vi "CAN_Send Diag Message.vi"(0 "Write Session in":refnum<k21>, 1 "Read Session in":refnum<k21>, 2 "Parttype ref":refnum<vi>, 3 "ODX File Path":path=path "C:/LegacyApp/DB_0CA_7100_4M0_0004_73710BVW3710/DB_0CA_7100_4M0_0004_73710BVW3710/DB_0CA_7100_4M0_0004_73710BVW3710.odx", 4 "Tx Msg":u8[](array[numeric])=[2, 26, 156, 255, 255, 255, 255, 255] format="%02x", 5 "error in (no error)":errorcluster, 6 "Enum":T2=enum."Get Calibration Status", 7 "Download CAL Progress":refnum<vi>, 10 "Postion":u16=3, 11 "Download CAL Time":refnum<vi>, 12 "Autotest":bool, 14 "ECU Info in":T1, 17 "Tester":refnum<k21>) -> (13 "Response Good?":bool, 15 "ECU Info":T1, 16 "pass?":bool, 18 "TxRx Data":string[][](array[string]), 19 "error out":errorcluster)   [LabVIEW 2014]
uses:
  Diagnostic Message.ctl
  typedefs/parttype.ctl
  <vilib>/xnet/xnet.llb/XNET Frame CAN.ctl
  <vilib>/xnet/xnet.llb/XNET Frame Type CAN.ctl
  CAN Communication VI's/Typedefs/Select Session.ctl
  typedefs/All Motions.ctl
  <vilib>/xnet/xnet.llb/XNET Write (Frame CAN).vi
  <vilib>/xnet/xnet.llb/XNET Read (Frame CAN).vi
panel:
  out "Rx Message":u8[](array[numeric]) format="%02x"
  out "Error String Out":string
  in  "Tx Arbitration Id":u32=402391172 format="%.0x"
  out "Part Number":string
  out "Vehicle Type":string
  out "SW level":string
  out "Calibrated":bool
  out "HW level":string
  out "CAL level":string
  out "Boot level":string
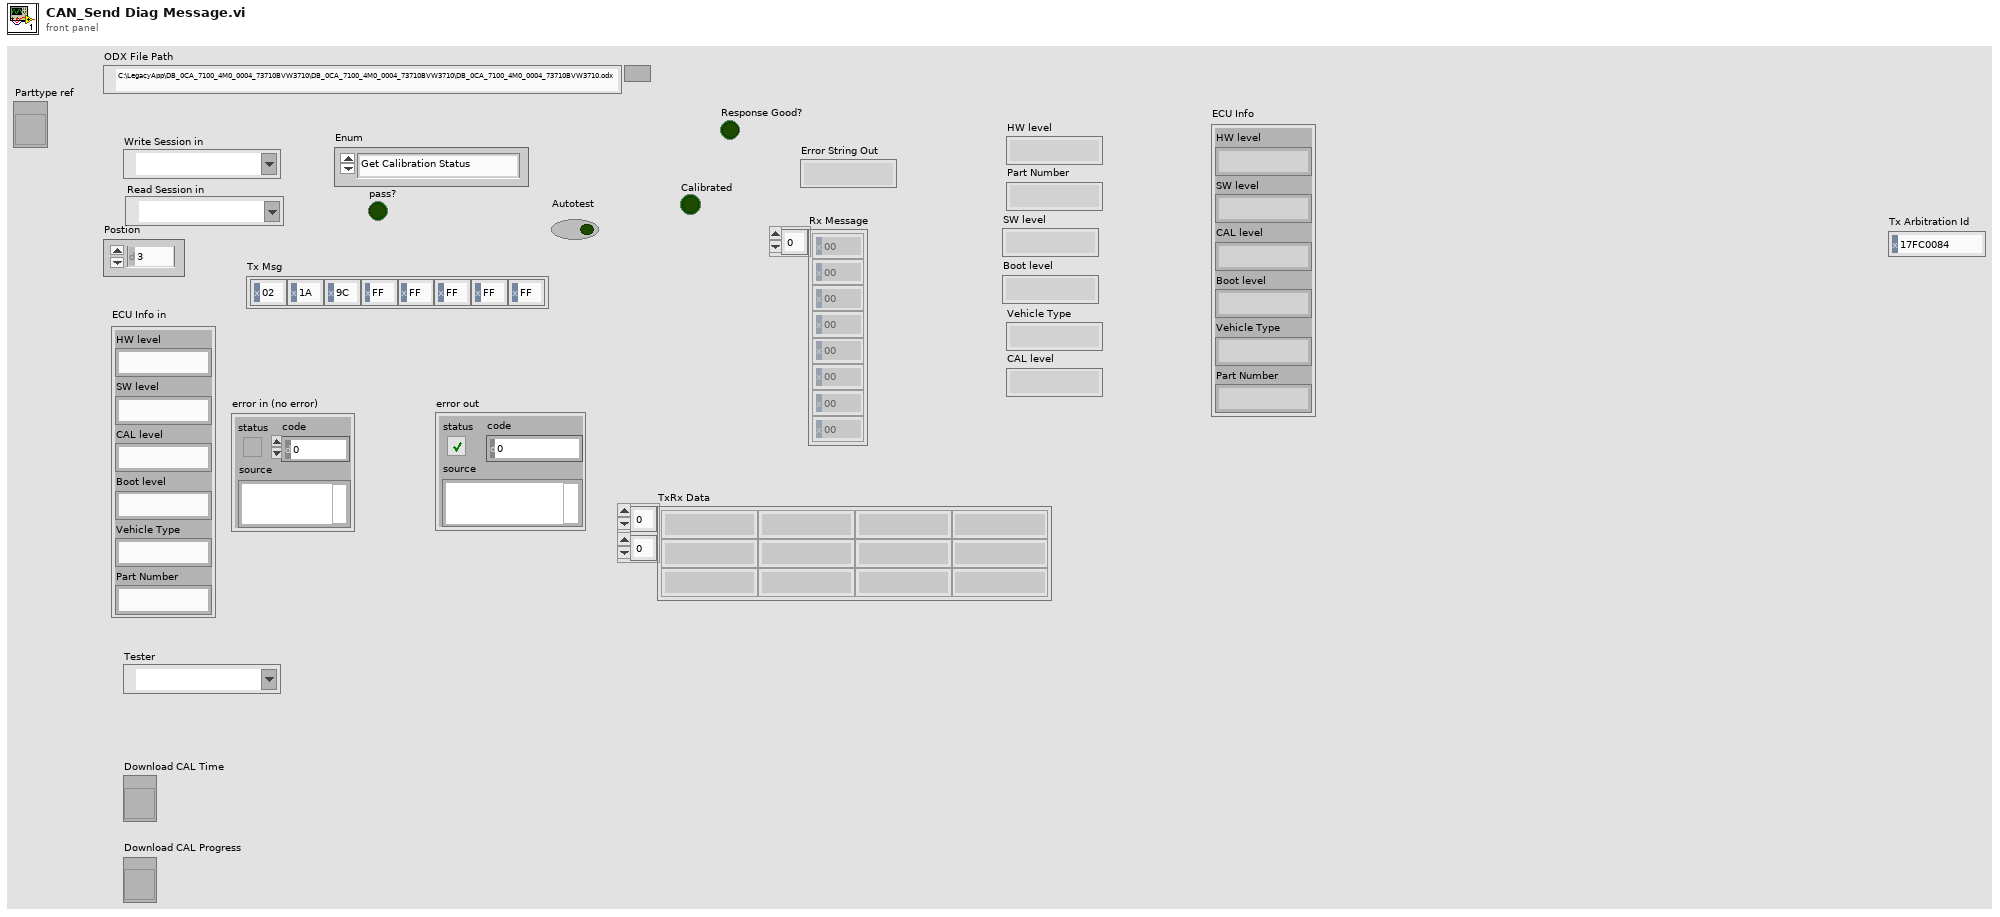
[diagram p1: front panel]
types:
  T1 = cluster{"HW level":string, "SW level":string, "CAL level":string, "Boot level":string, "Vehicle Type":string, "Part Number":string}
  T2 = typedef "Diagnostic Message.ctl" = enum16{"User Select", "Get User Multi-Frame", "Diag Session Prog", "Diag Session Ext", "Diag Session EOL", "Diag Session Default", "Diag Session Dev", "Read Active Session", "Read HW", "Read SW", "Read Part Number", "Learn Start Glass", "Learn Start Rollo", "Get Calibration Status", "Read SW CAL Boot", "Go to Position", "Get Parametric Mode Status", "Enable Parametric Mode", "Disable Parametric Mode", "Enable Production Mode", "Disable Production Mode", "Reset ECU", "Go to Slide Close", "Go to Slide Open", "Go to Vent Open", "Rollo Open", "Rollo Close", "Write Vehicle Type", "Read Vehicle Type", "Clear DTC", "Check Teach DTC", "Write Shop Code", "Download CAL", "Finish Flash", "Delete RP RF"}
  T3 = typedef "XNET Frame CAN.ctl" = cluster{"timestamp":timestamp, "payload":u8[], "identifier":u32, "type":T4, "extended?":bool, "echo?":bool}
  T4 = typedef "XNET Frame Type CAN.ctl" = u8
  T5 = typedef "Select Session.ctl" = enum16{"DefaultSession", "Development", "Extended", "EOL", "Programming"}
  T6 = typedef "All Motions.ctl" = enum16{"Idle", "Glass Teach", "Glass Slide Open", "Glass Slide Open 2", "Glass Slide Close", "Glass Slide Close 2", "Glass Vent Open", "Glass Vent Close", "Sunshade Teach", "Sunshade Teach 2", "Sunshade Open", "Sunshade Open 2", "Sunshade Close", "Sunshade Close 2", "Glass Slide Open Sunshade Open", "Glass Slide Open 2 Sunshade Open", "Glass Slide Open Sunshade Close", "Glass Slide Open 2 Sunshade Close", "Glass Slide Close Sunshade Open", "Glass Slide Close 2 Sunshade Open", "Glass Slide Close Sunshade Close", "Glass Slide Close 2 Sunshade Close", "Glass Vent Open Sunshade Open", "Glass Vent Open Sunshade Close", "Glass Vent Close Sunshade Open", "Glass Vent Close Sunshade Close", "Express Glass Slide Open", "Express Glass Slide Open 2", "Express Glass Slide Close", "Express Glass Slide Close 2", "Express Glass Vent Open", "Express Glass Vent Close", "Express Sunshade Open", "Express Sunshade Close", "Express Sunshade Open 2", "Express Sunshade Close 2", "Express Glass Slide Open Sunshade Open", "Express Glass Slide Open 2 Sunshade Open", "Express Glass Slide Open Sunshade Close", "Express Glass Slide Open 2 Sunshade Close", "Express Glass Slide Close Sunshade Open", "Express Glass Slide Close 2 Sunshade Open", "Express Glass Slide Close Sunshade Close", "Express Glass Slide Close 2 Sunshade Close", "Express Glass Vent Open Sunshade Open", "Express Glass Vent Open Sunshade Close", "Express Glass Vent Close Sunshade Open", "Express Glass Vent Close Sunshade Close", "Goto Position Glass", "Goto Position Sunshade"}
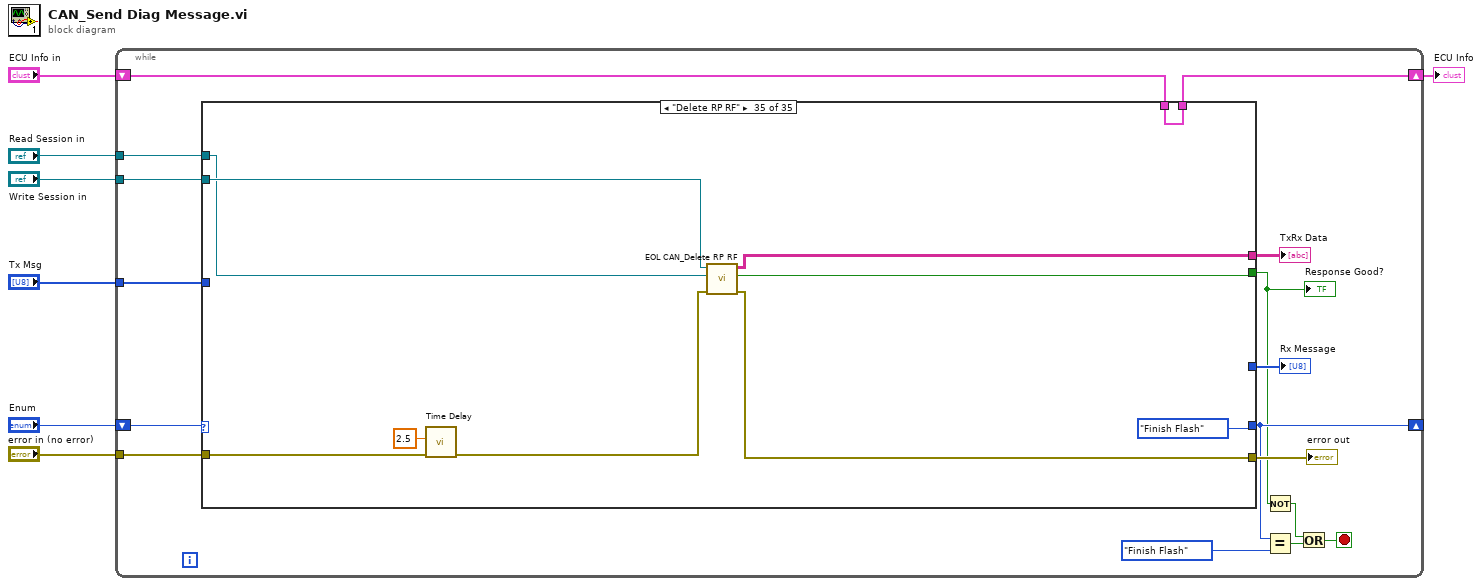
[diagram p0: block diagram]
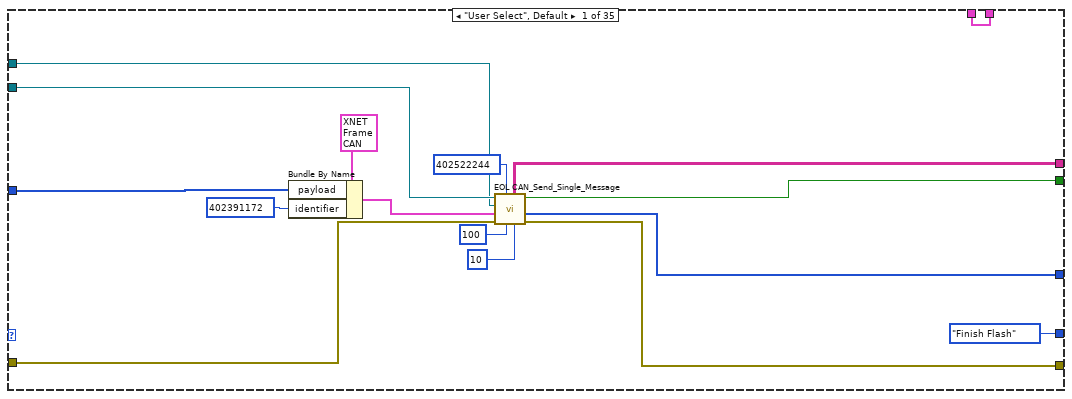
[diagram p2: hidden frame]
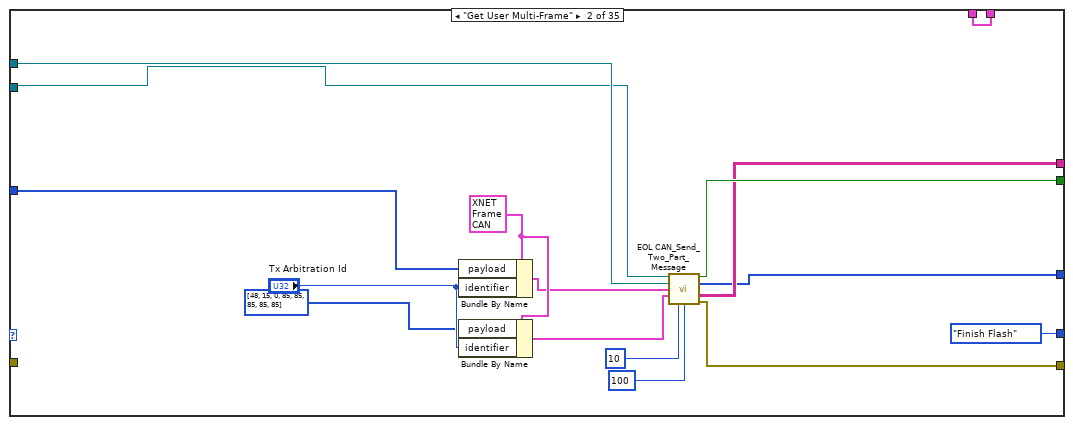
[diagram p3: hidden frame]
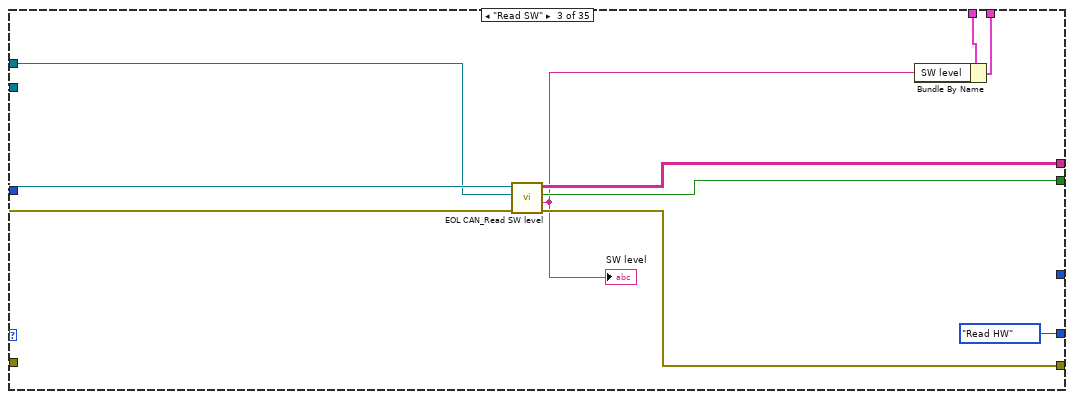
[diagram p4: hidden frame]
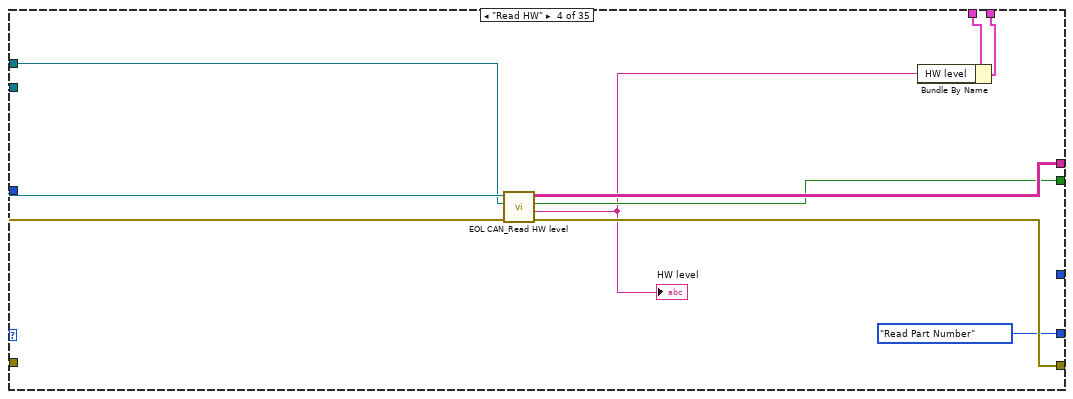
[diagram p5: hidden frame]
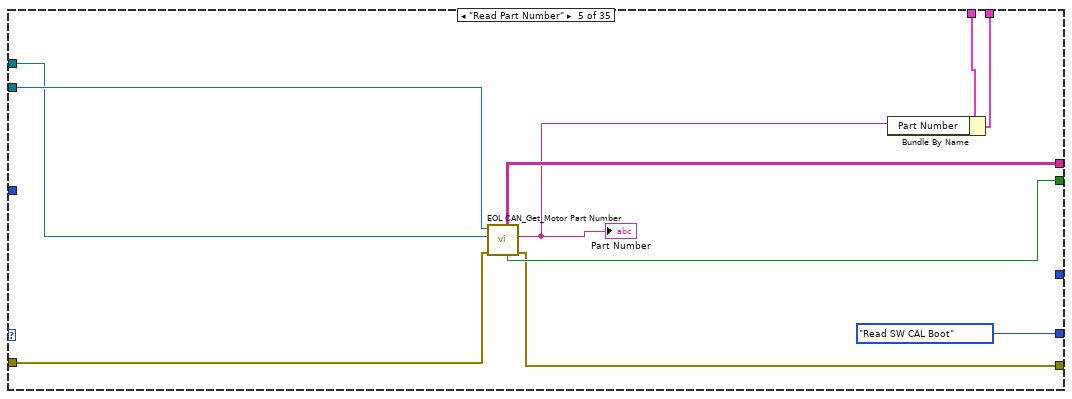
[diagram p6: hidden frame]
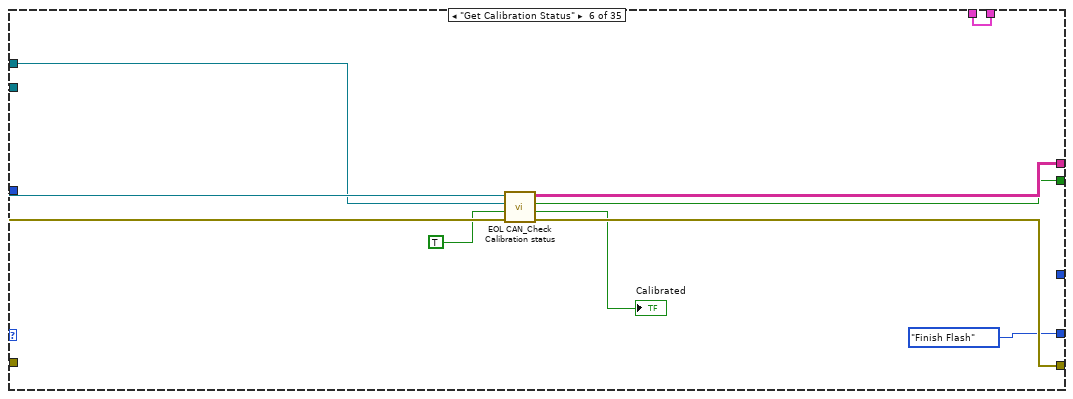
[diagram p7: hidden frame]
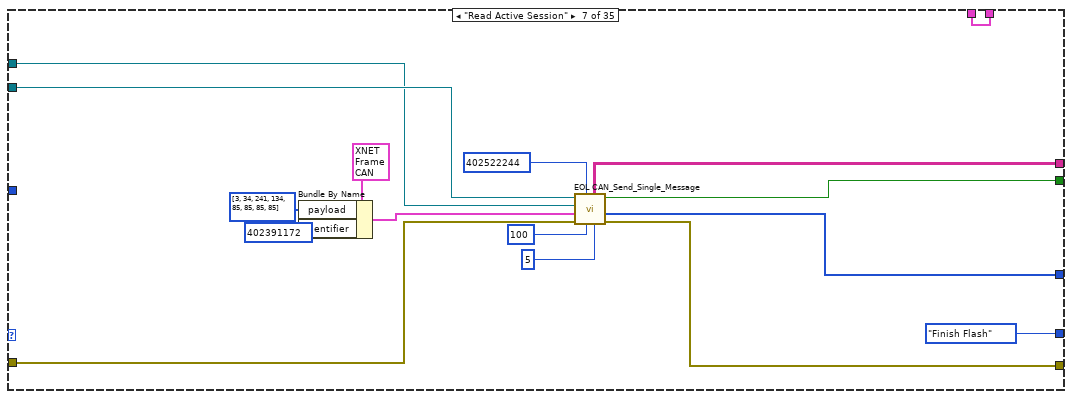
[diagram p8: hidden frame]
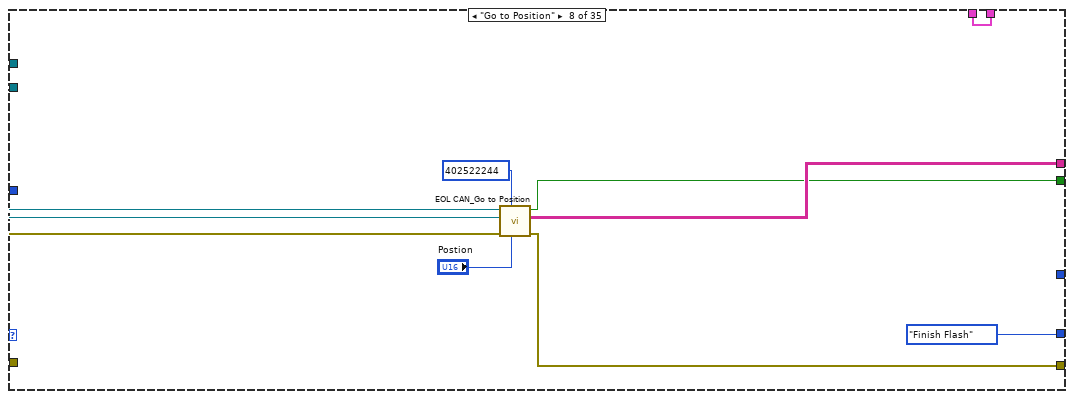
[diagram p9: hidden frame]
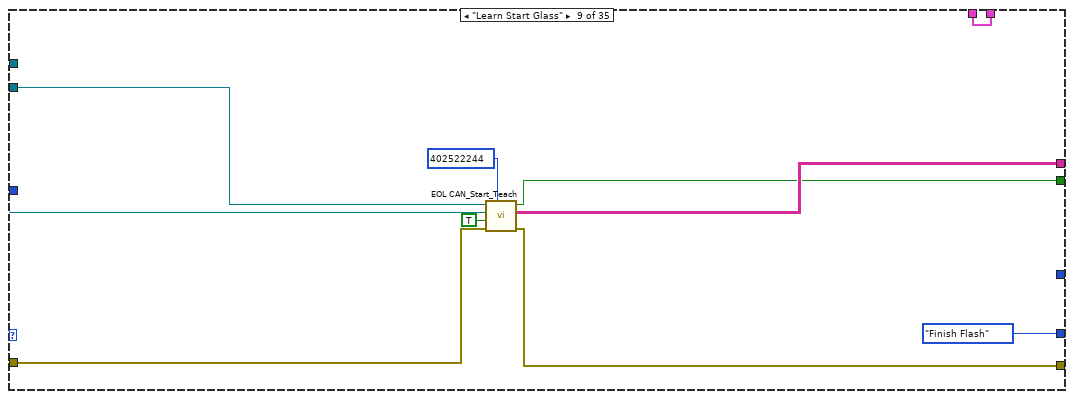
[diagram p10: hidden frame]
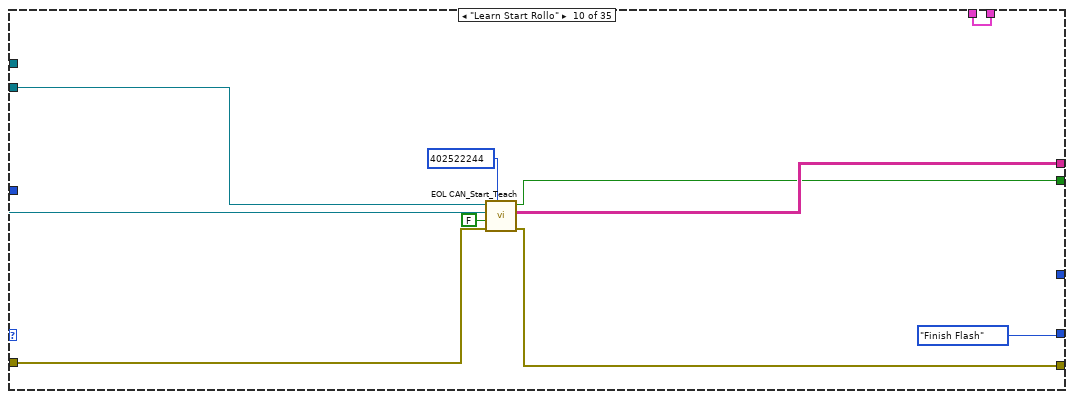
[diagram p11: hidden frame]
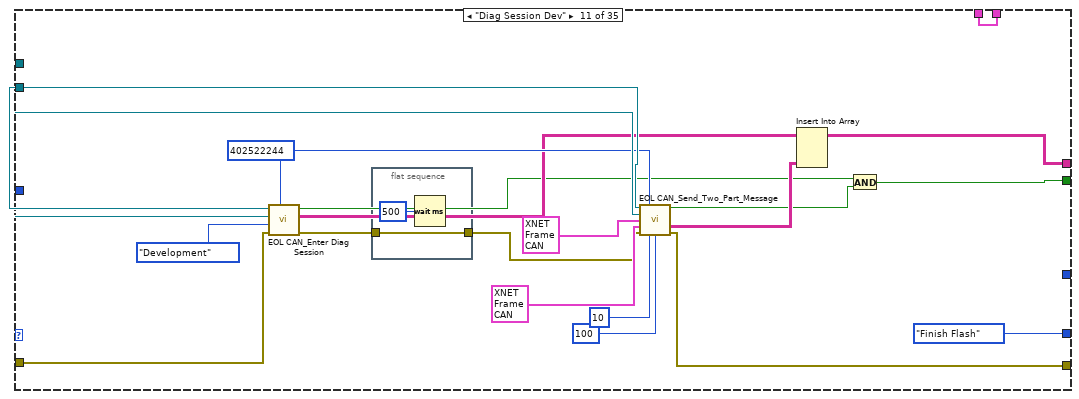
[diagram p12: hidden frame]
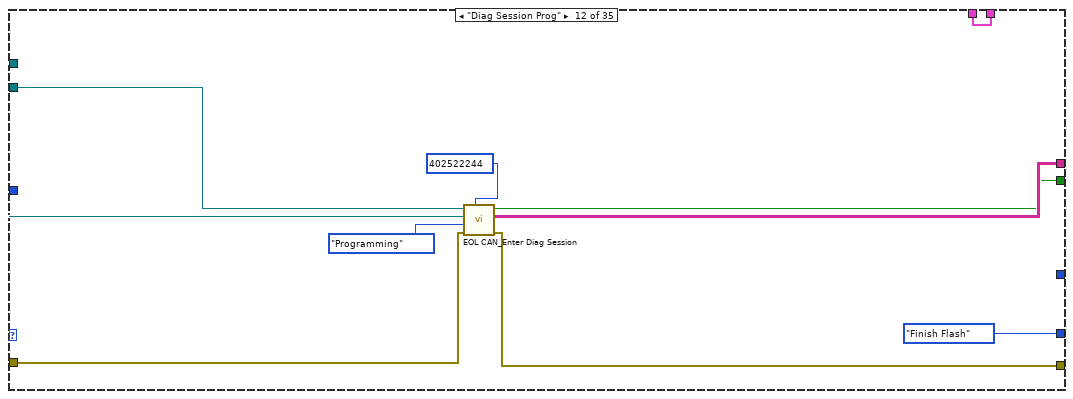
[diagram p13: hidden frame]
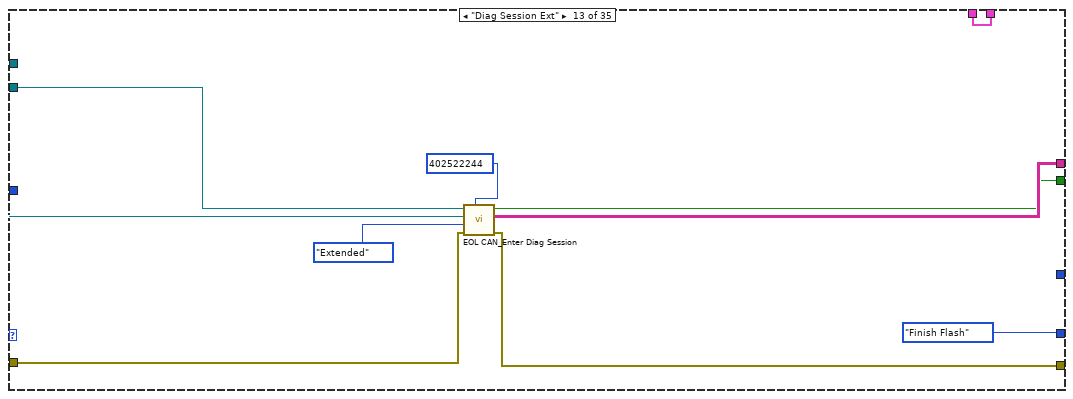
[diagram p14: hidden frame]
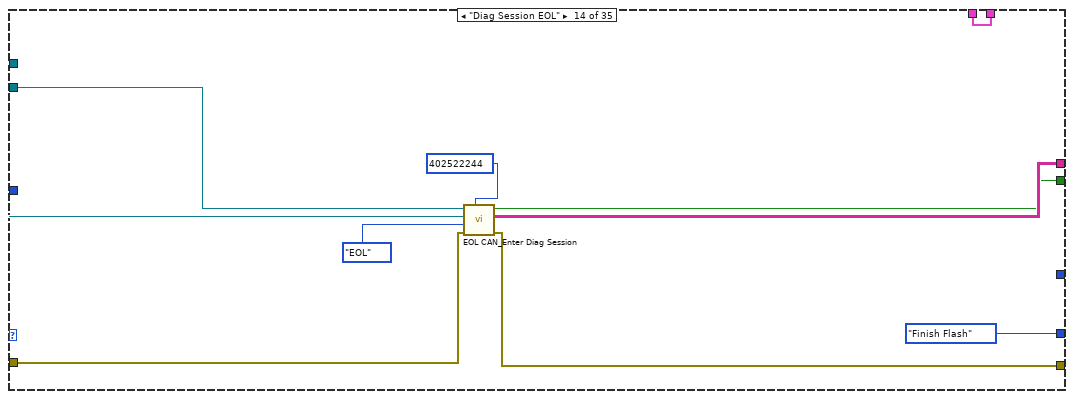
[diagram p15: hidden frame]
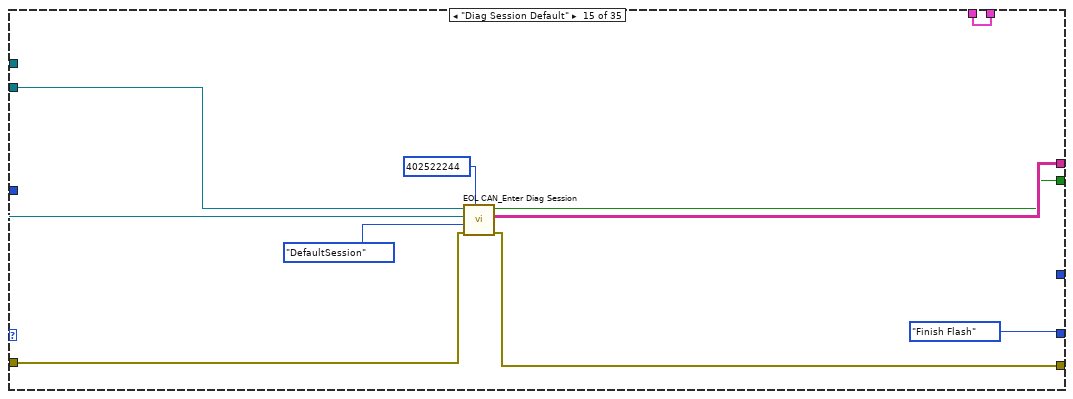
[diagram p16: hidden frame]
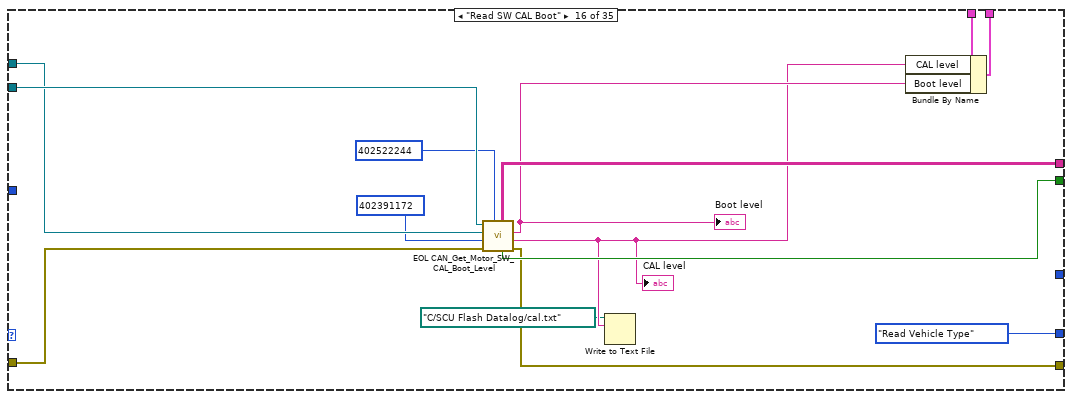
[diagram p17: hidden frame]
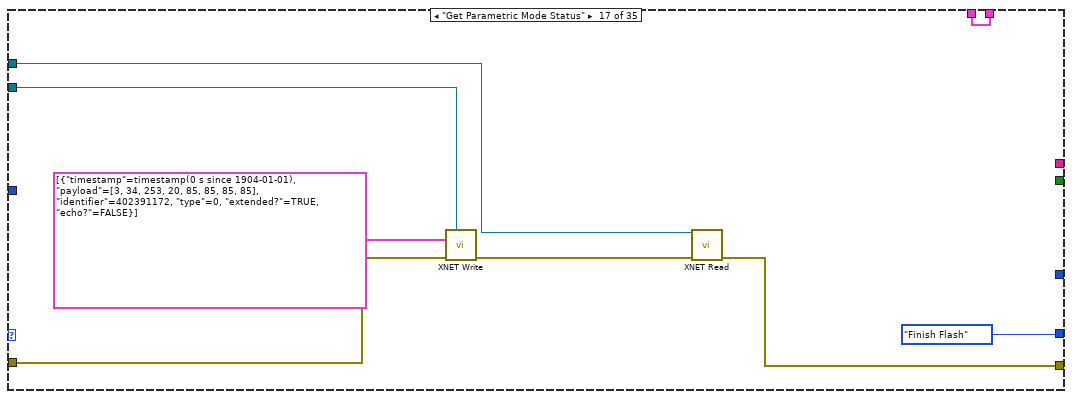
[diagram p18: hidden frame]
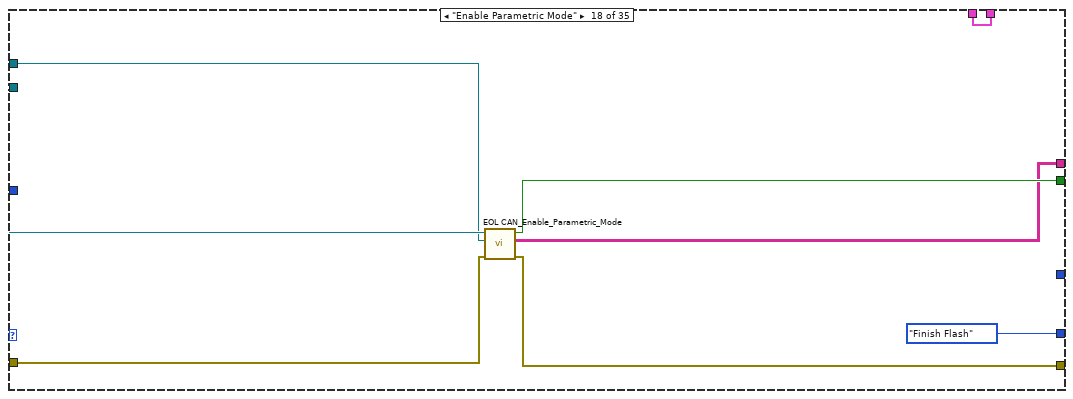
[diagram p19: hidden frame]
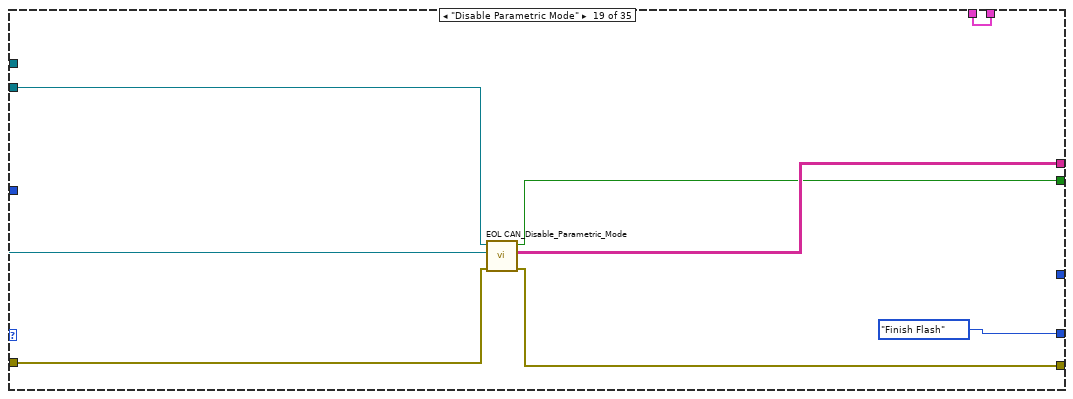
[diagram p20: hidden frame]
diagram:
  n1 = while {
    tunnel: "error in (no error)" -> [w23]
    tunnel: "Read Session in" -> [w21]
    tunnel: "Write Session in" -> [w20]
    shift-right: [w17] -> w3
    shift-left: "ECU Info in" -> [w16]
    tunnel: "Tx Msg" -> [w15]
    shift-right: [w10] -> _
    shift-left: "Enum" -> [w19]
    stop <- w13 stop-if-true
    n2 = case shown="\"Delete RP RF\"" w19 {
      tunnel: w21 -> [w38 w47 w60 w70 w83 w94 w110 w118 w129 w139 w157 w167 w177 w187 w197 w215 w223 w231 w236 w247 w255 w264 w274 w284 w294 w304 w314 w318 w326 w350 w365 w372 w382 _ w411]
      tunnel: w20 -> [w39 w46 w61 w71 w84 w95 w111 w119 w130 w140 w159 w168 w178 w188 w198 w216 w225 w232 w237 w248 w256 w265 w275 w285 w295 w305 w315 w319 w327 w351 w364 w373 w384 _ w412]
      tunnel: w23 -> [w37 _ w65 w75 w85 w93 w109 w121 w131 w141 w161 w173 w183 w193 w203 w217 w224 w233 w241 w249 w257 w266 w276 w286 w296 w306 w316 _ _ _ w366 w374 w383 w402 w406]
      tunnel: [w36 w42 w64 w74 w80 w92 w108 w120 w127 w137 w158 w172 w182 w192 w202 w210 w220 w228 w240 w244 w252 w260 w270 w280 w290 w300 w310 w322 w330 errorcluster {"status"=FALSE, "code"=0, "source"=""} ("error IO") w359 w371 w381 w402 w408] -> w22
      tunnel: [w35 w43 w63 w73 w82 w91 w107 w116 w126 w136 w151 w171 w181 w191 w201 w212 _ w229 w239 w245 w253 w262 w271 w281 w291 w301 w311 w323 w331 w346 w361 w369 _ _ w410] -> w18
      tunnel: [w34 w44 w62 w72 w81 w88 w106 w115 w125 w135 w148 w170 w180 w190 w200 w211 _ w230 w238 w246 w254 w261 w272 w282 w292 w302 w312 w321 w329 w336 w360 w370 _ _ w409] -> w9
      tunnel: [w33 w41 _ _ _ _ w103 _ _ _ _ _ _ _ _ _ _ _ _ _ _ _ _ _ _ _ _ w320 w328 _ _ _ _ _ _] -> w14
      tunnel: [w26 w55 w58 w67 w78 w87 w97 w113 w124 w134 w143 w165 w175 w185 w195 w208 w219 w227 w235 w243 w251 w259 w268 w278 w288 w298 w308 w324 w332 w354 w357 w368 w376 w403 w413] -> w17
      tunnel: w16 -> [w26 w55 w59 w68 w77 w87 w97 w113 w124 w134 w143 w165 w175 w185 w195 w209 w219 w227 w235 w243 w251 w259 w268 w278 w288 w298 w308 w324 w332 w354 w358 w368 w376 w403 w413]
      tunnel: w15 -> [w25 w45 _ _ _ _ _ _ _ _ _ _ _ _ _ _ _ _ _ _ _ _ _ _ _ _ _ _ _ _ _ _ _ _ _]
      tunnel: [Diagnostic_Message."Finish Flash" ("Enum") Diagnostic_Message."Finish Flash" ("Enum") Diagnostic_Message."Read HW" ("Enum") Diagnostic_Message."Read Part Number" ("Enum") Diagnostic_Message."Read SW CAL Boot" ("Enum") Diagnostic_Message."Finish Flash" ("Enum") Diagnostic_Message."Finish Flash" ("Enum") Diagnostic_Message."Finish Flash" ("Enum") Diagnostic_Message."Finish Flash" ("Enum") Diagnostic_Message."Finish Flash" ("Enum") Diagnostic_Message."Finish Flash" ("Enum") Diagnostic_Message."Finish Flash" ("Enum") Diagnostic_Message."Finish Flash" ("Enum") Diagnostic_Message."Finish Flash" ("Enum") Diagnostic_Message."Finish Flash" ("Enum") Diagnostic_Message."Read Vehicle Type" ("Enum") Diagnostic_Message."Finish Flash" ("Enum") Diagnostic_Message."Finish Flash" ("Enum") Diagnostic_Message."Finish Flash" ("Enum") Diagnostic_Message."Delete RP RF" ("Enum") Diagnostic_Message."Finish Flash" ("Enum") Diagnostic_Message."Finish Flash" ("Enum") Diagnostic_Message."Finish Flash" ("Enum") Diagnostic_Message."Finish Flash" ("Enum") Diagnostic_Message."Finish Flash" ("Enum") Diagnostic_Message."Finish Flash" ("Enum") Diagnostic_Message."Finish Flash" ("Enum") Diagnostic_Message."Finish Flash" ("Enum") Diagnostic_Message."Finish Flash" ("Enum") w339 Diagnostic_Message."Enable Production Mode" ("Enum") Diagnostic_Message."Finish Flash" ("Enum") Diagnostic_Message."Finish Flash" ("Enum") Diagnostic_Message."Finish Flash" ("Enum") Diagnostic_Message."Finish Flash" ("Enum")] -> w10
      frame "User Select", Default {
        n3 = Bundle By Name(cluster=T3 {"timestamp"=timestamp(0 s since 1904-01-01), "payload"=[2, 39, 3, 85, 85, 85, 85, 85], "identifier"=402391172, "type"=0, "extended?"=TRUE, "echo?"=FALSE} ("Tx CAN frame"), "payload"=w25, "identifier"=u32 402391172) -> (w31:T3)
        n4 = call "EOL CAN_Send_Single_Message.vi"("Retries"=10, "Msg Wait Time"=u32 100, "Rx Arbitration Id"=u32 402522244, "Error in"=w37, "Tx CAN frame"=w31, "Read Session in"=w38, "Write Session in"=w39) -> ("Error out"=w36:errorcluster, "Rx Message"=w33:u8[], "Response Good?"=w34:bool, "TxRx Data"=w35:string[][])  [unwired: 1 out]
      }
      frame "Get User Multi-Frame" {
        w49 = T3 {"timestamp"=timestamp(0 s since 1904-01-01), "payload"=[2, 39, 3, 85, 85, 85, 85, 85], "identifier"=402391172, "type"=0, "extended?"=TRUE, "echo?"=FALSE} ("Tx CAN frame 1")
        n5 = Bundle By Name(cluster=w49, "payload"=w45, "identifier"="Tx Arbitration Id") -> (w48:T3)
        n6 = Bundle By Name(cluster=w49, "payload"=u8[] [48, 15, 0, 85, 85, 85, 85, 85] ("Transmit Data"), "identifier"="Tx Arbitration Id") -> (w50:T3)
        n7 = call "EOL CAN_Send_Two_Part_Message.vi"("Write Session in"=w46, "Read Session in"=w47, "Tx CAN frame 1"=w48, "Tx CAN frame 2"=w50, "Retries"=10, "Msg Wait Time"=u32 100) -> ("Response Good?"=w44:bool, "Rx Data"=w41:u8[], "TxRx Data"=w43:string[][], "error out"=w42:errorcluster)  [unwired: 6 in]
      }
      frame "Read SW" {
        n8 = call "EOL CAN_Read SW level.vi"("error in (no error)"=w65, "Read Session in"=w60, "Write Session in"=w61) -> ("error out"=w64:errorcluster, "SW level"=w57:string, "Response Good?"=w62:bool, "TxRx Data"=w63:string[][])  [unwired: 5 in]
        "SW level" <- w57
        n9 = Bundle By Name(cluster=w59, "SW level"=w57) -> (w58:T1)
      }
      frame "Read HW" {
        n10 = call "EOL CAN_Read HW level.vi"("error in (no error)"=w75, "Read Session in"=w70, "Write Session in"=w71) -> ("error out"=w74:errorcluster, "HW level"=w69:string, "Response Good?"=w72:bool, "TxRx Data"=w73:string[][])  [unwired: 5 in]
        "HW level" <- w69
        n11 = Bundle By Name(cluster=w68, "HW level"=w69) -> (w67:T1)
      }
      frame "Read Part Number" {
        n12 = call "EOL CAN_Get_Motor Part Number.vi"("error in (no error)"=w85, "Read Session in"=w83, "Write Session in"=w84) -> ("error out"=w80:errorcluster, "Part Number"=w79:string, "Response Good?"=w81:bool, "TxRx Data"=w82:string[][])  [unwired: 5 in]
        "Part Number" <- w79
        n13 = Bundle By Name(cluster=w77, "Part Number"=w79) -> (w78:T1)
      }
      frame "Get Calibration Status" {
        n14 = call "EOL CAN_Check Calibration status.vi"("error in (no error)"=w93, "Glass?"=TRUE, "Read Session in"=w94, "Write Session in"=w95) -> ("error out"=w92:errorcluster, "Calibrated"=→"Calibrated":bool, "Response Good?"=w88:bool, "TxRx Data"=w91:string[][])  [unwired: 4 in]
      }
      frame "Read Active Session" {
        n15 = Bundle By Name(cluster=T3 {"timestamp"=timestamp(0 s since 1904-01-01), "payload"=[2, 39, 3, 85, 85, 85, 85, 85], "identifier"=402391172, "type"=0, "extended?"=TRUE, "echo?"=FALSE} ("Tx CAN frame"), "payload"=u8[] [3, 34, 241, 134, 85, 85, 85, 85], "identifier"=u32 402391172) -> (w100:T3)
        n16 = call "EOL CAN_Send_Single_Message.vi"("Retries"=5, "Msg Wait Time"=u32 100, "Rx Arbitration Id"=u32 402522244, "Error in"=w109, "Tx CAN frame"=w100, "Read Session in"=w110, "Write Session in"=w111) -> ("Error out"=w108:errorcluster, "Rx Message"=w103:u8[], "Response Good?"=w106:bool, "TxRx Data"=w107:string[][])  [unwired: 1 out]
      }
      frame "Go to Position" {
        n17 = call "EOL CAN_Go to Position.vi"("Postion"="Postion", "Rx Arbitration Id"=u32 402522244, "Error in"=w121, "Read Session in"=w118, "Write Session in"=w119) -> ("Error out"=w120:errorcluster, "TxRx Data"=w116:string[][], "Response Good?"=w115:bool)  [unwired: 4 in]
      }
      frame "Learn Start Glass" {
        n18 = call "EOL CAN_Start_Teach.vi"("Rx Arbitration Id"=u32 402522244, "Error in"=w131, "Glass?"=TRUE, "Read Session in"=w129, "Write Session in"=w130) -> ("Error out"=w127:errorcluster, "TxRx Data"=w126:string[][], "Response Good?"=w125:bool)  [unwired: 4 in]
      }
      frame "Learn Start Rollo" {
        n19 = call "EOL CAN_Start_Teach.vi"("Rx Arbitration Id"=u32 402522244, "Error in"=w141, "Glass?"=FALSE, "Read Session in"=w139, "Write Session in"=w140) -> ("Error out"=w137:errorcluster, "TxRx Data"=w136:string[][], "Response Good?"=w135:bool)  [unwired: 4 in]
      }
      frame "Diag Session Dev" {
        w156 = u32 402522244 ("Rx Arbitration Id")
        n20 = call "EOL CAN_Enter Diag Session.vi"("Rx Arbitration Id"=w156, "Error in"=w161, "Session"=Select_Session."Development", "Read Session in"=w157, "Write Session in"=w159) -> ("Error out"=w147:errorcluster, "TxRx Data"=w153:string[][], "Response Good?"=w149:bool)  [unwired: 4 in]
        n21 = flat-sequence {
          tunnel: w147 -> [w162]
          tunnel: [w162] -> w146
          frame #0 {
            n22 = Wait (ms)(milliseconds to wait=u32 500) -> ()  [unwired: 1 out]
          }
        }
        n23 = call "EOL CAN_Send_Two_Part_Message.vi"("Write Session in"=w159, "Rx Arbitration Id"=w156, "Read Session in"=w157, "Tx CAN frame 1"=T3 {"timestamp"=timestamp(0 s since 1904-01-01), "payload"=[3, 34, 254, 253, 85, 85, 85, 85], "identifier"=402391172, "type"=8, "extended?"=TRUE, "echo?"=FALSE}, "Tx CAN frame 2"=T3 {"timestamp"=timestamp(0 s since 1904-01-01), "payload"=[48, 15, 0, 85, 85, 85, 85, 85], "identifier"=402391172, "type"=8, "extended?"=TRUE, "echo?"=FALSE}, "error in (no error)"=w146, "Retries"=10, "Msg Wait Time"=u32 100) -> ("Response Good?"=w150:bool, "TxRx Data"=w152:string[][], "error out"=w158:errorcluster)  [unwired: 4 in, 1 out]
        n24 = Insert Into Array(array=w153, new element=w152) -> (w151:string[][])  [unwired: 2 in]
        n25 = And(x=w149, y=w150) -> (x .and. y?=w148:bool)
      }
      frame "Diag Session Prog" {
        n26 = call "EOL CAN_Enter Diag Session.vi"("Rx Arbitration Id"=u32 402522244, "Error in"=w173, "Session"=Select_Session."Programming", "Read Session in"=w167, "Write Session in"=w168) -> ("Error out"=w172:errorcluster, "TxRx Data"=w171:string[][], "Response Good?"=w170:bool)  [unwired: 4 in]
      }
      frame "Diag Session Ext" {
        n27 = call "EOL CAN_Enter Diag Session.vi"("Rx Arbitration Id"=u32 402522244, "Error in"=w183, "Session"=Select_Session."Extended", "Read Session in"=w177, "Write Session in"=w178) -> ("Error out"=w182:errorcluster, "TxRx Data"=w181:string[][], "Response Good?"=w180:bool)  [unwired: 4 in]
      }
      frame "Diag Session EOL" {
        n28 = call "EOL CAN_Enter Diag Session.vi"("Rx Arbitration Id"=u32 402522244, "Error in"=w193, "Session"=Select_Session."EOL", "Read Session in"=w187, "Write Session in"=w188) -> ("Error out"=w192:errorcluster, "TxRx Data"=w191:string[][], "Response Good?"=w190:bool)  [unwired: 4 in]
      }
      frame "Diag Session Default" {
        n29 = call "EOL CAN_Enter Diag Session.vi"("Rx Arbitration Id"=u32 402522244, "Error in"=w203, "Session"=Select_Session."DefaultSession", "Read Session in"=w197, "Write Session in"=w198) -> ("Error out"=w202:errorcluster, "TxRx Data"=w201:string[][], "Response Good?"=w200:bool)  [unwired: 4 in]
      }
      frame "Read SW CAL Boot" {
        n30 = call "EOL CAN_Get_Motor_SW_CAL_Boot_Level.vi"("Rx Arbitration Id"=u32 402522244, "error in (no error)"=w217, "Tx Arbitration Id"=u32 402391172 ("identifier"), "Read Session in"=w215, "Write Session in"=w216) -> ("error out"=w210:errorcluster, "CAL level"=w205:string, "Boot level"=w207:string, "Response Good?"=w211:bool, "TxRx Data"=w212:string[][])  [unwired: 1 in, 1 out]
        "Boot level" <- w207
        "CAL level" <- w205
        n31 = Write to Text File(file (use dialog)=path "C:/SCU Flash Datalog/cal.txt", text=w205) -> ()  [unwired: 2 in, 3 out]
        n32 = Bundle By Name(cluster=w209, "CAL level"=w205, "Boot level"=w207) -> (w208:T1)
      }
      frame "Get Parametric Mode Status" {
        n33 = call-poly <vilib>:"XNET Write.vi"("session in"=w225, "data"=T3[] [{"timestamp"=timestamp(0 s since 1904-01-01), "payload"=[3, 34, 253, 20, 85, 85, 85, 85], "identifier"=402391172, "type"=0, "extended?"=TRUE, "echo?"=FALSE}] ("Frame to Send 2"), "error in (no error)"=w224) -> ("error out"=w221:errorcluster)  [unwired: 11 in, 1 out]
        n34 = call-poly <vilib>:"XNET Read.vi"("session in"=w223, "error in (no error)"=w221) -> ("error out"=w220:errorcluster)  [unwired: 10 in, 3 out]
      }
      frame "Enable Parametric Mode" {
        n35 = call "EOL CAN_Enable_Parametric_Mode.vi"("Error in"=w233, "Read Session in"=w231, "Write Session in"=w232) -> ("Error out"=w228:errorcluster, "debug log"=w229:string[][], "Response Good?"=w230:bool)  [unwired: 6 in]
      }
      frame "Disable Parametric Mode" {
        n36 = call "EOL CAN_Disable_Parametric_Mode.vi"("Error in"=w241, "Read Session in"=w236, "Write Session in"=w237) -> ("Error out"=w240:errorcluster, "debug log"=w239:string[][], "Response Good?"=w238:bool)  [unwired: 6 in]
      }
      frame "Enable Production Mode" {
        n37 = call "EOL CAN_Enable_Production_Mode.vi"("Error in"=w249, "Read Session in"=w247, "Write Session in"=w248) -> ("Error out"=w244:errorcluster, "debug log"=w245:string[][], "Response Good?"=w246:bool)  [unwired: 6 in]
      }
      frame "Disable Production Mode" {
        n38 = call "EOL CAN_Disable_Production_Mode.vi"("Error in"=w257, "Read Session in"=w255, "Write Session in"=w256) -> ("Error out"=w252:errorcluster, "debug log"=w253:string[][], "Response Good?"=w254:bool)  [unwired: 6 in]
      }
      frame "Reset ECU" {
        n39 = call "EOL CAN_Reset ECU.vi"("Rx Arbitration Id"=u32 402522244, "Error in"=w266, "Read Session in"=w264, "Write Session in"=w265) -> ("Error out"=w260:errorcluster, "Response Good?"=w261:bool, "TxRx Data"=w262:string[][])  [unwired: 5 in]
      }
      frame "Go to Slide Close" {
        n40 = call "EOL CAN_Target Motion.vi"("Rx Arbitration Id"=u32 402522244, "Error in"=w276, "All Motions"=All_Motions."Glass Slide Close", "Read Session in"=w274, "Write Session in"=w275) -> ("Error out"=w270:errorcluster, "TxRx Data"=w271:string[][], "Response Good?"=w272:bool)  [unwired: 4 in]
      }
      frame "Go to Slide Open" {
        n41 = call "EOL CAN_Target Motion.vi"("Rx Arbitration Id"=u32 402522244, "Error in"=w286, "All Motions"=All_Motions."Glass Slide Open", "Read Session in"=w284, "Write Session in"=w285) -> ("Error out"=w280:errorcluster, "TxRx Data"=w281:string[][], "Response Good?"=w282:bool)  [unwired: 4 in]
      }
      frame "Go to Vent Open" {
        n42 = call "EOL CAN_Target Motion.vi"("Rx Arbitration Id"=u32 402522244, "Error in"=w296, "All Motions"=All_Motions."Glass Vent Open", "Read Session in"=w294, "Write Session in"=w295) -> ("Error out"=w290:errorcluster, "TxRx Data"=w291:string[][], "Response Good?"=w292:bool)  [unwired: 4 in]
      }
      frame "Rollo Open" {
        n43 = call "EOL CAN_Target Motion.vi"("Rx Arbitration Id"=u32 402522244, "Error in"=w306, "All Motions"=All_Motions."Sunshade Open", "Read Session in"=w304, "Write Session in"=w305) -> ("Error out"=w300:errorcluster, "TxRx Data"=w301:string[][], "Response Good?"=w302:bool)  [unwired: 4 in]
      }
      frame "Rollo Close" {
        n44 = call "EOL CAN_Target Motion.vi"("Rx Arbitration Id"=u32 402522244, "Error in"=w316, "All Motions"=All_Motions."Sunshade Close", "Read Session in"=w314, "Write Session in"=w315) -> ("Error out"=w310:errorcluster, "TxRx Data"=w311:string[][], "Response Good?"=w312:bool)  [unwired: 4 in]
      }
      frame "Write Vehicle Type" {
        n45 = call "EOL CAN_Write Vehicle Type.vi"("Read Session in"=w318, "Write Session in"=w319) -> ("error out"=w322:errorcluster, "Rx Message"=w320:u8[], "Response Good?"=w321:bool, "Array"=w323:string[][])  [unwired: 6 in]
      }
      frame "Write Shop Code" {
        n46 = call "EOL CAN_Write Repair Shop Code.vi"("Read Session in"=w326, "Write Session in"=w327) -> ("error out"=w330:errorcluster, "Rx Message"=w328:u8[], "Response Good?"=w329:bool, "TxRxData"=w331:string[][])  [unwired: 6 in]
      }
      frame "Download CAL" {
        n47 = call "EOL CAN_Download CAL.vi"("DSC Write Session in"=w351, "Tester"="Tester", "Download CAL Time"="Download CAL Time", "Read Session in"=w350, "Parttype ref"="Parttype ref", "Glass?"=TRUE, "ODX File Path"="ODX File Path", "Download CAL Progress"="Download CAL Progress") -> ("Response Good?"=w336:bool, "TxRx Data"=w346:string[][], "Error String Out"=→"Error String Out":string, "fail"=w337:bool)  [unwired: 4 in]
        n48 = Not(x=w337) -> (.not. x?=w335:bool)
        n49 = Select(t=Diagnostic_Message."Read SW" ("Enum"), s="Autotest", f=Diagnostic_Message."Finish Flash" ("Enum")) -> (s? t:f=w340:T2)
        n50 = And(x=w336, y=w335) -> (x .and. y?=→"pass?":bool)
        n51 = Select(t=w340, s=w336, f=Diagnostic_Message."Finish Flash") -> (s? t:f=w339:T2)
      }
      frame "Read Vehicle Type" {
        n52 = call "EOL CAN_Get Vehicle type.vi"("Rx Arbitration Id"=u32 402522244, "error in (no error)"=w366, "Tx Arbitration Id"=u32 402391172, "Read Session in"=w365, "Write Session in"=w364) -> ("error out"=w359:errorcluster, "Vehicle Type"=w356:string, "Response Good?"=w360:bool, "TxRx Data"=w361:string[][])  [unwired: 3 in]
        "Vehicle Type" <- w356
        n53 = Bundle By Name(cluster=w358, "Vehicle Type"=w356) -> (w357:T1)
      }
      frame "Clear DTC" {
        n54 = call "EOL CAN_Clear_DTC's.vi"("Error in"=w374, "Read Session in"=w372, "Write Session in"=w373) -> ("Error out"=w371:errorcluster, "TxRx Data"=w369:string[][], "Response Good?"=w370:bool)  [unwired: 6 in]
      }
      frame "Check Teach DTC" {
        n55 = stacked-sequence {
          tunnel: w384 -> [w392 w400]
          tunnel: w383 -> [w391 w399]
          tunnel: [w389 _] -> w380
          tunnel: w382 -> [w390 w398]
          tunnel: [w388 _] -> w378
          tunnel: [_ w397] -> w377
          tunnel: [_ w396] -> w379
          frame #0 {
            n56 = call-poly <vilib>:"XNET Write.vi"("session in"=w392, "data"=T3[] [{"timestamp"=timestamp(0 s since 1904-01-01), "payload"=[2, 16, 79, 85, 85, 85, 85, 85], "identifier"=402391172, "type"=0, "extended?"=TRUE, "echo?"=FALSE}] ("Frame to Send 2"), "error in (no error)"=w391) -> ("error out"=w386:errorcluster)  [unwired: 11 in, 1 out]
            n57 = call "Time Delay22"("error in (no error)"=w386, "Delay Time (s)"=0.05) -> ("error out"=w385:errorcluster)  [unwired: 9 in]
            n58 = call-poly <vilib>:"XNET Read.vi"("session in"=w390, "error in (no error)"=w385) -> ("data"=w388:T3[], "error out"=w389:errorcluster)  [unwired: 10 in, 2 out]
          }
          frame #1 {
            n59 = call-poly <vilib>:"XNET Write.vi"("session in"=w400, "data"=T3[] [{"timestamp"=timestamp(0 s since 1904-01-01), "payload"=[3, 34, 241, 134, 85, 85, 85, 85], "identifier"=402391172, "type"=0, "extended?"=TRUE, "echo?"=FALSE}] ("Frame to Send 2"), "error in (no error)"=w399) -> ("error out"=w395:errorcluster)  [unwired: 11 in, 1 out]
            n60 = call-poly <vilib>:"XNET Read.vi"("session in"=w398, "error in (no error)"=w395) -> ("data"=w397:T3[], "error out"=w396:errorcluster)  [unwired: 10 in, 2 out]
          }
        }
        n61 = Build Array (concatenate)(w378, w377) -> ()  [unwired: 1 out]
        n62 = Merge Errors(w380, w379) -> (w381:errorcluster)
      }
      frame "Finish Flash" {
      }
      frame "Delete RP RF" {
        n63 = call "Time Delay"("error in (no error)"=w406, "Delay Time (s)"=2.5) -> ("error out"=w405:errorcluster)  [unwired: 9 in]
        n64 = call "EOL CAN_Delete RP RF.vi"("error in (no error)"=w405, "Read Session in"=w411, "Write Session in"=w412) -> ("error out"=w408:errorcluster, "Response Good?"=w409:bool, "TxRx Data"=w410:string[][])  [unwired: 6 in]
      }
    }
    "error out" <- w22
    "TxRx Data" <- w18
    "Response Good?" <- w9
    "Rx Message" <- w14
    n65 = Not(x=w9) -> (.not. x?=w8:bool)
    n66 = Equal?(x=w10, y=Diagnostic_Message."Finish Flash" ("Enum")) -> (x = y?=w11:bool)
    n67 = Or(x=w8, y=w11) -> (x .or. y?=w13:bool)
  }
  "ECU Info" <- w3
